vi "Add New Blocks.vi"(8 "error in (no error)":errorcluster, 9 "# to Add":i32=2, 10 "Grid":refnum<data-value>, 11 "Board in":refnum<class "Board.lvclass">) -> (0 "error out":errorcluster, 1 "No Busy":bool, 2 "New Shapes":refnum<data-value>[](array[refnum]), 3 "Board in 2":refnum<class "Board.lvclass">)   [LabVIEW 2016]
uses:
  Board/Board.lvclass
  <vilib>/LIEF/Forms/Shape/Shape.lvclass
  Board/Board.lvclass/Board.ctl
  Block/Block.lvclass
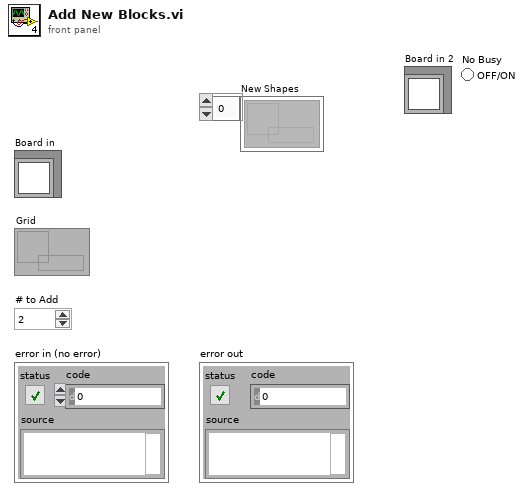
[diagram p1: front panel]
types:
  T1 = cluster{"number: 0 to 1":dbl, "number: 0 to 1":dbl}
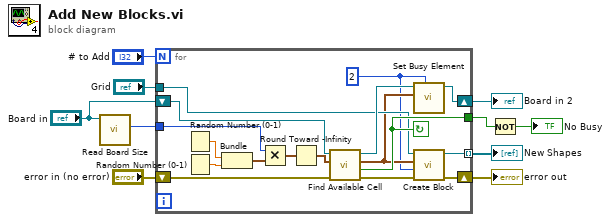
[diagram p0: block diagram]
diagram:
  n1 = call "Read Board Size.vi"("Board in"="Board in") -> ("Board Size"=w3:u16)  [unwired: 8 in, 2 out]
  n2 = for {
    N: "# to Add" -> [_]
    tunnel: "Grid" -> [w13]
    tunnel: [w15] -> w7 mode=indexing
    shift-right: [w23] -> w5
    shift-left: "Board in" -> [w22]
    tunnel: w3 -> [w19]
    shift-right: [w17] -> w10
    shift-left: "error in (no error)" -> [w18]
    tunnel: [w16] -> w2
    stop <- w16 continue-if-true
    w11 = u32 2 ("Text")
    n3 = Random Number (0-1)() -> (number: 0 to 1=w24:dbl)
    n4 = Random Number (0-1)() -> (number: 0 to 1=w27:dbl)
    n5 = Bundle("number: 0 to 1"=w24, "number: 0 to 1"=w27) -> (w26:T1)  [unwired: 1 in]
    n6 = Multiply(x=w19, y=w26) -> (x*y=w25:T1)
    n7 = Round Toward -Infinity(1:w25) -> (0:w20:T1)
    n8 = call "Find Available Cell.vi"("error in (no error)"=w18, "Indexes"=w20, "Board in"=w22) -> ("error out"=w14:errorcluster, "Free Cell Found"=w16:bool, "Available Indexes"=w12:cluster{i32, i32}, "Board out"=w21:refnum<class "Board.lvclass">)  [unwired: 5 in]
    n9 = call "Set Busy Element.vi"("New Block"=w11, "Indexes"=w12, "Board in"=w21) -> ("Board out"=w23:refnum<class "Board.lvclass">)  [unwired: 7 in, 1 out]
    n10 = call "Create Block.vi"("error in (no error)"=w14, "Value"=w11, "Available Indexes"=w12, "Grid"=w13) -> ("error out"=w17:errorcluster, "New Block"=w15:refnum<data-value>)  [unwired: 6 in]
  }
  "error out" <- w10
  "New Shapes" <- w7
  "Board in 2" <- w5
  n11 = Not(x=w2) -> (.not. x?=→"No Busy":bool)
